vi "HRV_Analysis.vi"(8 "Frame Length":i32=100, 10 "Sample Rate":dbl=500.0 format="%#_13g", 11 "PPG_Data":dbl[](array[numeric])) -> (2 "PPI":dbl, 3 "PRV% (VLF, LF, HF)":dbl[](array[numeric]))   [LabVIEW 2014]
uses:
  <vilib>/Analysis/NI_AAL_SigProc.lvlib
  <vilib>/Analysis/NI_AALBase.lvlib
  <vilib>/Analysis/NI_AALPro.lvlib
  <vilib>/gmath/NI_Gmath.lvlib
panel:
  out "SDNN":dbl
  out "Dominant_Distribution":dbl
  out "BPM":dbl
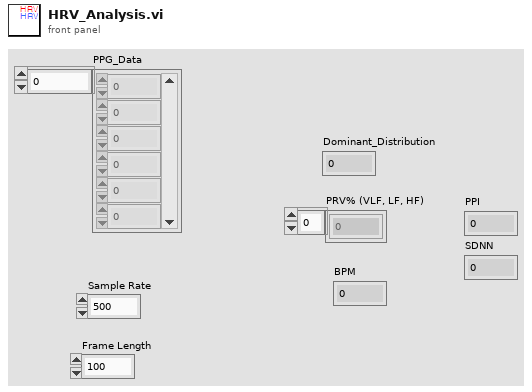
[diagram p1: front panel]
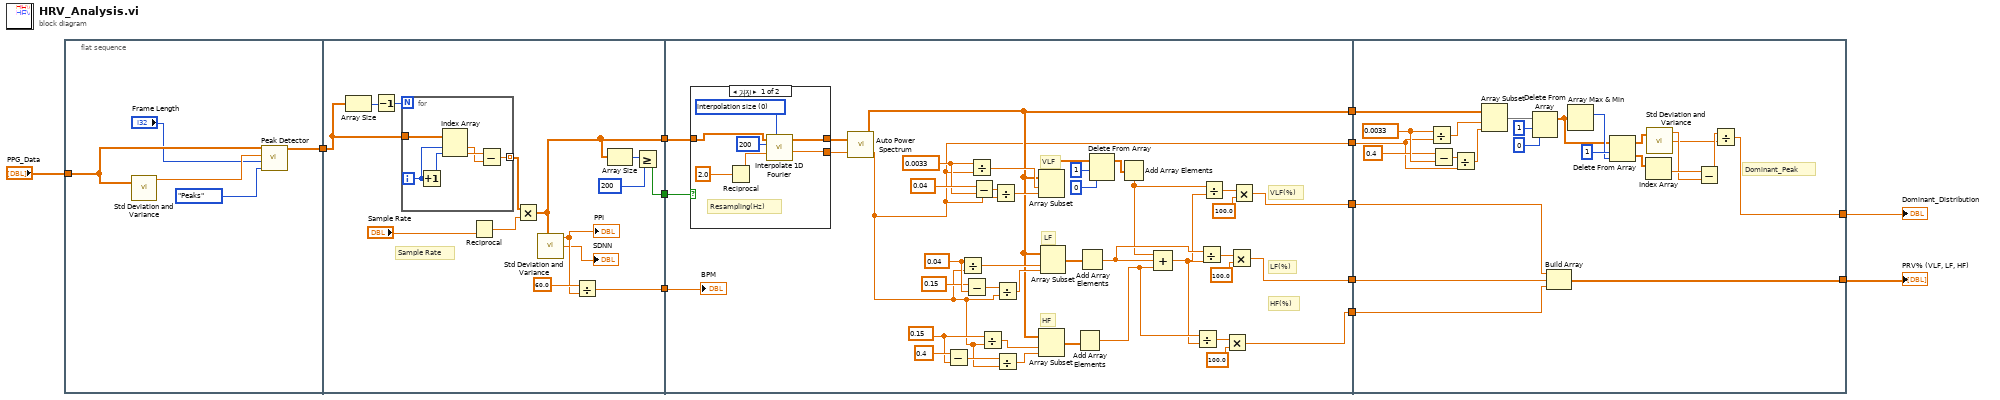
[diagram p0: block diagram]
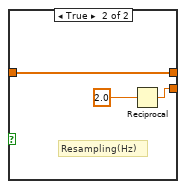
[diagram p2: hidden frame]
diagram:
  n1 = flat-sequence {
    tunnel: [w16] -> w12
    tunnel: "PPG_Data" -> [w14]
    tunnel: w12 -> [w29]
    tunnel: [w24] -> w11
    tunnel: [w21] -> w10
    tunnel: [w19] -> w2
    tunnel: w11 -> [w52]
    tunnel: [w54] -> w9
    tunnel: [w53] -> w8
    tunnel: [w42] -> w7
    tunnel: [w41] -> w6
    tunnel: [w40] -> w5
    tunnel: w10 -> [w39]
    tunnel: w2 -> [w38]
    tunnel: w9 -> [w112]
    tunnel: w8 -> [w108]
    tunnel: [w97] -> w3
    tunnel: w7 -> [w96]
    tunnel: w6 -> [w95]
    tunnel: w5 -> [w94]
    tunnel: [w93] -> w4
    frame #0 {
      n2 = call <vilib>:"Std Deviation and Variance.vi"("X"=w14) -> ("mean"=w15:dbl)  [unwired: 1 in, 2 out]
      n3 = call <vilib>:"Peak Detector.vi"("peaks/valleys"=enum32{"Peaks", "Valleys"}."Peaks", "width"="Frame Length", "threshold"=w15, "X"=w14) -> ("Locations"=w16:dbl[])  [unwired: 3 in, 4 out]
    }
    frame #1 {
      # "Sample Rate"
      n4 = Array Size(array=w29) -> (size(s)=w31:i32)
      n5 = Decrement(x=w31) -> (x-1=w30:i32)
      n6 = for {
        N: w30 -> [_]
        tunnel: w29 -> [w37]
        tunnel: [w32] -> w28 mode=indexing
        i -> [w35]
        n7 = Increment(x=w35) -> (x+1=w36:i32)
        n8 = Index Array(array=w37, index #1=w35, index #2=w36) -> (element #1=w33:dbl, element #2=w34:dbl)
        n9 = Subtract(x=w34, y=w33) -> (x-y=w32:dbl)
      }
      n10 = Reciprocal(x="Sample Rate") -> (1/x=w27:dbl)
      n11 = Multiply(x=w28, y=w27) -> (x*y=w24:dbl[])
      n12 = call <vilib>:"Std Deviation and Variance.vi"("X"=w24) -> ("mean"=w20:dbl, "standard deviation"=→"SDNN":dbl)  [unwired: 1 in, 1 out]
      "PPI" <- w20
      n13 = Divide(x=60.0, y=w20) -> (x/y=w19:dbl)
      n14 = Array Size(array=w24) -> (size(s)=w23:i32)
      n15 = Greater Or Equal?(x=w23, y=200) -> (x >= y?=w21:bool)
    }
    frame #2 {
      w66 = 0.0033 ("x")
      w71 = 0.15 ("x")
      w77 = 0.04 ("x")
      # "VLF(%)"
      # "LF(%)"
      # "HF(%)"
      # "VLF"
      # "HF"
      # "LF"
      n16 = case shown="거짓" w39 {
        tunnel: w52 -> [w81 w87]
        tunnel: [w80 w86] -> w51
        tunnel: [w79 w87] -> w50
        frame False {
          w83 = u16 0 items=["interpolation size", "interpolation factor"] ("type")
          # "Resampling(Hz)"
          n17 = Reciprocal(x=2.0 ("Resampling(Hz)")) -> (1/x=w84:dbl)
          n18 = call <vilib>:"Interpolate 1D Fourier.vi"("type"=w83, "dt in"=w84, "n"=200, "X"=w81) -> ("dt out"=w80:dbl, "Y"=w79:dbl[])  [unwired: 4 in, 2 out]
        }
        frame True {
          # "Resampling(Hz)"
          n19 = Reciprocal(x=2.0 ("Resampling(Hz)")) -> (1/x=w86:dbl)
        }
      }
      n20 = call <vilib>:"Auto Power Spectrum.vi"("dt"=w51, "Signal (V)"=w50) -> ("df"=w53:dbl, "Power Spectrum (V^2 rms)"=w54:dbl[])
      n21 = Subtract(x=0.4, y=w71) -> (x-y=w73:dbl)
      n22 = Divide(x=w77, y=w53) -> (x/y=w78:dbl)
      n23 = Subtract(x=0.15, y=w77) -> (x-y=w75:dbl)
      n24 = Divide(x=w66, y=w53) -> (x/y=w65:dbl)
      n25 = Subtract(x=0.04, y=w66) -> (x-y=w68:dbl)
      n26 = Divide(x=w71, y=w53) -> (x/y=w70:dbl)
      n27 = Divide(x=w68, y=w53) -> (x/y=w64:dbl)
      n28 = Divide(x=w75, y=w53) -> (x/y=w74:dbl)
      n29 = Divide(x=w73, y=w53) -> (x/y=w69:dbl)
      n30 = Array Subset(array=w54, index=w65, length=w64) -> (w56:dbl[])
      n31 = Array Subset(array=w54, index=w70, length=w69) -> (w62:dbl[])
      n32 = Array Subset(array=w54, index=w78, length=w74) -> (w63:dbl[])
      n33 = Add Array Elements(numeric array=w62) -> (sum=w61:dbl)
      n34 = Add Array Elements(numeric array=w63) -> (sum=w47:dbl)
      n35 = Delete From Array(array=w56, length=1 ("길이"), index=0 ("인덱스")) -> (array with subset deleted=w55:dbl[])  [unwired: 1 out]
      n36 = Add Array Elements(numeric array=w55) -> (sum=w43:dbl)
      n37 = Compound Arithmetic op=ADD(w43, w47, w61) -> (w44:dbl)
      n38 = Divide(x=w61, y=w44) -> (x/y=w60:dbl)
      n39 = Divide(x=w47, y=w44) -> (x/y=w48:dbl)
      n40 = Divide(x=w43, y=w44) -> (x/y=w46:dbl)
      n41 = Multiply(x=w60, y=100.0) -> (x*y=w40:dbl)
      n42 = Multiply(x=w48, y=100.0) -> (x*y=w41:dbl)
      n43 = Multiply(x=w46, y=100.0) -> (x*y=w42:dbl)
      "BPM" <- w38
    }
    frame #3 {
      w111 = 0.0033 ("x")
      # "Dominant_Peak"
      n44 = Divide(x=w111, y=w108) -> (x/y=w107:dbl)
      n45 = Subtract(x=0.4, y=w111) -> (x-y=w109:dbl)
      n46 = Divide(x=w109, y=w108) -> (x/y=w106:dbl)
      n47 = Array Subset(array=w112, index=w107, length=w106) -> (w103:dbl[])
      n48 = Delete From Array(array=w103, length=1 ("길이"), index=0 ("인덱스")) -> (array with subset deleted=w91:dbl[])  [unwired: 1 out]
      n49 = Build Array(w96, w95, w94) -> (w93:dbl[])
      n50 = Array Max & Min(array=w91) -> (max index (indices)=w101:i32)  [unwired: 3 out]
      n51 = Delete From Array(array=w91, length=1 ("길이"), index=w101) -> (deleted portion=w98:dbl[], array with subset deleted=w99:dbl[])
      n52 = Index Array(array=w98) -> (element=w100:dbl)  [unwired: 1 in]
      n53 = call <vilib>:"Std Deviation and Variance.vi"("X"=w99) -> ("mean"=w92:dbl, "standard deviation"=w89:dbl)  [unwired: 1 in, 1 out]
      n54 = Subtract(x=w100, y=w92) -> (x-y=w90:dbl)
      n55 = Divide(x=w90, y=w89) -> (x/y=w97:dbl)
    }
  }
  "PRV% (VLF, LF, HF)" <- w4
  "Dominant_Distribution" <- w3
